vi "Read Module Menu Name.vi"(8 "error in":errorcluster, 11 "Simple Sequencer TBM editor node in":refnum<class "Simple Sequencer TBM editor node.lvclass">) -> (0 "error out":errorcluster, 2 "Menu Name":string, 3 "Simple Sequencer TBM editor node out":refnum<class "Simple Sequencer TBM editor node.lvclass">)   [LabVIEW 2014, in "Simple Sequencer TBM editor node.lvclass"]
uses:
  Simple Sequencer TBM editor node.lvclass
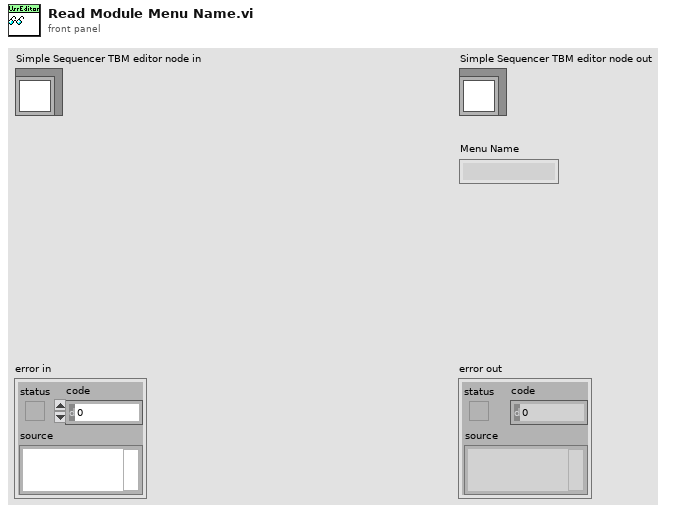
[diagram p1: front panel]
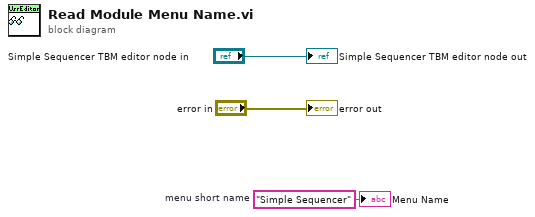
[diagram p0: block diagram]
diagram:
  w1 = "Simple Sequencer"  # menu short name
  "error out" <- "error in"
  "Simple Sequencer TBM editor node out" <- "Simple Sequencer TBM editor node in"
  "Menu Name" <- w1
